vi "Test Method Description Reset on Test Start.vi"(8 "error in (no error)":errorcluster, 11 "Result Model Result Recording Test in":refnum<class "Result Model Result Recording Test.lvclass">) -> (0 "error out":errorcluster, 3 "Result Model Result Recording Test out":refnum<class "Result Model Result Recording Test.lvclass">)   [LabVIEW 2020, in "Result Model Result Recording Test.lvclass"]
uses:
  Result Model Result Recording Test.lvclass
  C:/Program Files (x86)/National Instruments/LabVIEW 2020/vi.lib/Astemes/LUnit/Test Case.lvclass
  Result/Result.ctl
  Result/Status.ctl
  Result/Type.ctl
  <vilib>/Astemes/LUnit/Test Case.lvclass/Test Case.ctl
  ae2c71b8-32bb-49d1-8500-0119bfec74ff.vi
  <vilib>/Astemes/LUnit/Palette/Pass.vi
  <vilib>/Astemes/LUnit/Palette/Fail.vi
  <vilib>/Astemes/LUnit/Compare Variants.vi
  <vilib>/Astemes/LUnit/Describe Comparison.vi
  <vilib>/Astemes/LUnit/Set Assertion Type.vi
  <vilib>/Astemes/LUnit/Add test result.vi
  <vilib>/Astemes/LUnit/Variant to string.vi
  <vilib>/Astemes/LUnit/LUnit Record Assertion Result.vi
  <vilib>/Astemes/LUnit/LUnit Aggregate Assertion Results.vi
  <vilib>/Astemes/LUnit/Method Result/LUnit Merge Status.vi
  <vilib>/Astemes/LUnit/LUnit Concatenate result strings.vi
  <vilib>/Utility/Data Type/Get Type Information.vi
  <vilib>/Utility/LVClass/Get LV Class Name.vi
  Result Model/Result Model.lvclass
  Result/Result.lvlib
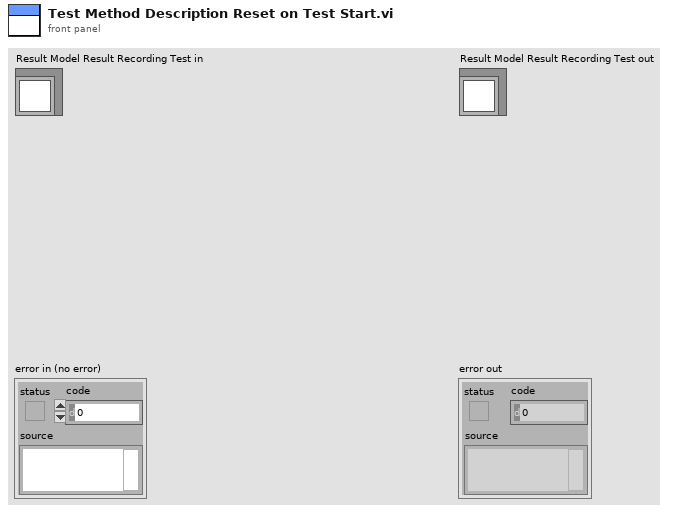
[diagram p1: front panel]
types:
  T1 = typedef "Result.lvlib/Result.ctl" = cluster{"Name":string, "Message":string, "Description":string, "Status":T2, "Result Type":T3, "Execution Time":dbl}
  T2 = typedef "Result.lvlib/Status.ctl" = enum16{"", "Passed", "Failed", "Error", "Skipped", "Setup Error", "Broken", "Teardown Error"}
  T3 = typedef "Result.lvlib/Type.ctl" = enum16{"Method", "Case", "Suite", "Pass", "Fail", "Skip", "Pass if", "Fail if", "Pass if Error", "Fail if Error", "Pass if Equal", "Fail if Equal"}
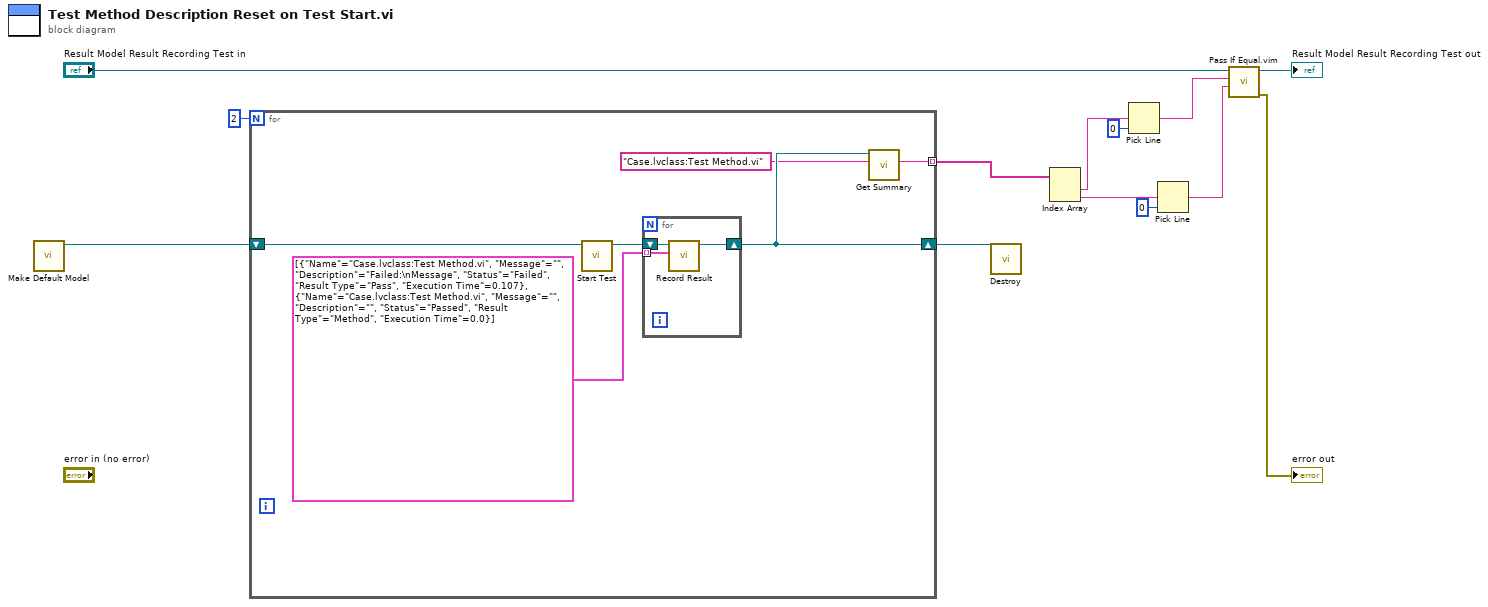
[diagram p0: block diagram]
diagram:
  n1 = call "Make Default Model.vi"() -> ("Result Model out"=w13:refnum<class "Result Model.lvclass">)  [unwired: 10 in, 1 out]
  n2 = for {
    N: 2 -> [_]
    shift-right: [w16] -> w8
    shift-left: w13 -> [w19]
    tunnel: [w15] -> w7 mode=indexing
    n3 = call "Start Test.vi"("Result Model In"=w19) -> ("Result Model Out"=w17:refnum<class "Result Model.lvclass">)  [unwired: 10 in]
    n4 = for {
      tunnel: T1[] [{"Name"="Case.lvclass:Test Method.vi", "Message"="", "Description"="Failed:\nMessage", "Status"=enum."Failed", "Result Type"=enum."Pass", "Execution Time"=0.107}, {"Name"="Case.lvclass:Test Method.vi", "Message"="", "Description"="", "Status"=enum."Passed", "Result Type"=enum."Method", "Execution Time"=0.0}] ("Results") -> [w21] mode=indexing
      shift-right: [w20] -> w16
      shift-left: w17 -> [w22]
      n5 = call "Record Result.vi"("Results"=w21, "Result Model in"=w22) -> ("Result Model out"=w20:refnum<class "Result Model.lvclass">)  [unwired: 9 in]
    }
    n6 = call "Get Summary.vi"("Item"="Case.lvclass:Test Method.vi", "Result Model In"=w16) -> ("Summary"=w15:string)  [unwired: 9 in]
  }
  n7 = call "Destroy.vi"("Result Model in"=w8) -> ()  [unwired: 10 in, 1 out]
  n8 = Index Array(array=w7) -> (element #1=w5:string, element #2=w3:string)  [unwired: 2 in]
  n9 = Pick Line(multi-line string=w5, line index=0) -> (output string=w6:string)  [unwired: 1 in]
  n10 = Pick Line(multi-line string=w3, line index=0) -> (output string=w2:string)  [unwired: 1 in]
  n11 = call "Pass If Equal.vim"("Actual"=w2, "Expected"=w6, "LUnit Test Case In"="Result Model Result Recording Test in") -> ("error out"=→"error out":errorcluster, "LUnit Test Case Out"=→"Result Model Result Recording Test out":refnum<class "Result Model Result Recording Test.lvclass">)  [unwired: 7 in]
